vi "Is Instance.vi"(0 "object under test":refnum<class>, 2 "target class":refnum<class>) -> (4 "object is an instance of target class":bool)   [LabVIEW 2015, in "LV Exceptions v1.lvlib"]
doc: "Tests if Object Under Test is an instance of target class."
uses:
  LV Exceptions v1.lvlib
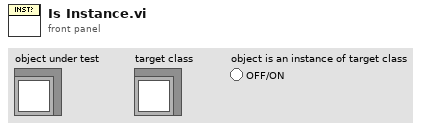
[diagram p1: front panel]
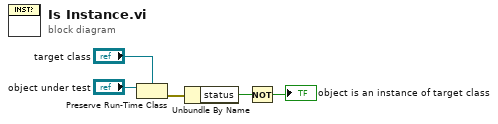
[diagram p0: block diagram]
diagram:
  n1 = Preserve Run-Time Class(object in="object under test", 2:"target class") -> (error out=w1:errorcluster)  [unwired: 1 in, 1 out]
  n2 = Unbundle By Name(w1) -> ("status"=w4:bool)
  n3 = Not(x=w4) -> (.not. x?=→"object is an instance of target class":bool)
